vi "new Simulation1553Type.vi"(8 "error in":errorcluster, 11 "errorInjection configuration":T1 {"errorMessages" items=["Tagged", "Any"]; "state" items=["Off", "On", "Once", "External"]}) -> (0 "error out":errorcluster, 3 "new Simulation1553Type":refnum<k24>)   [LabVIEW 2020, in "Ballard_1553_Hardware_ni.lvlib"]
uses:
  Ballard_1553_Hardware_ni.lvlib
  C:/Users/Administrator/Desktop/GIT/Ballard-MIL-STD-1553-Custom-Device/Source/System Explorer/SubVIs/Parse XML Ballard/1.2/BTIXML_SerDes.dll
  Ballard-MIL-STD-1553-Custom-Device/Source/System Explorer/SubVIs/Parse XML Ballard/1.2/BTIXML_SerDes.dll
  _typedefs/channel1553_errorInjection_type.ctl
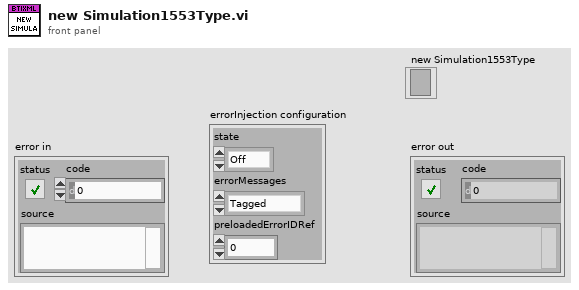
[diagram p1: front panel]
types:
  T1 = typedef "Ballard_1553_Hardware_ni.lvlib/channel1553_errorInjection_type.ctl" = cluster{"state":i32, "errorMessages":i32, "preloadedErrorIDRef":i32}
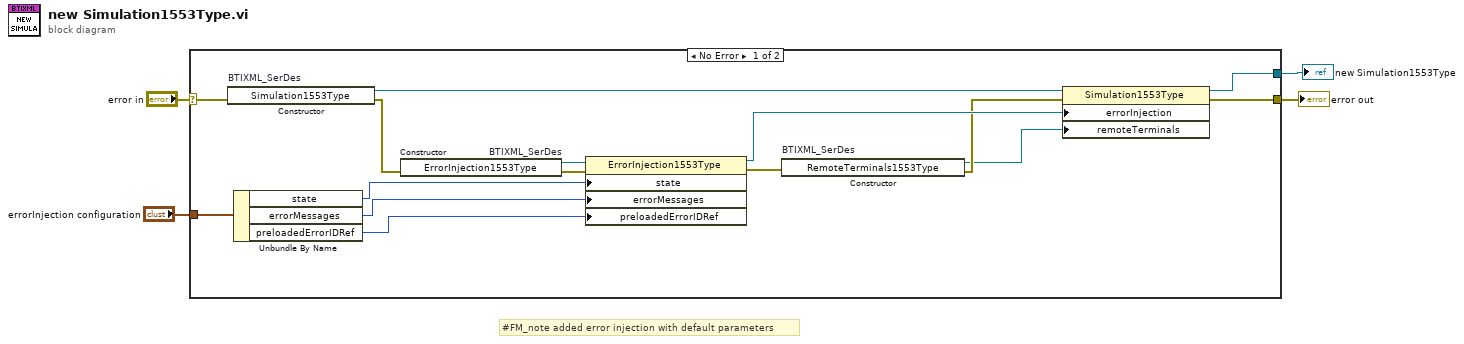
[diagram p0: block diagram]
diagram:
  # "#FM_note added error injection with default parameters"
  n1 = case shown="No Error" "error in" {
    selector: "error in" -> [w18 w20]
    tunnel: [w17 w20] -> w3
    tunnel: [w16 _] -> w1
    tunnel: "errorInjection configuration" -> [w12 _]
    frame No Error {
      n2 = constructor on="BTIXML_SerDes" class="Simulation1553Type"(error in=w18) -> (reference out=w19:refnum<k24>, error out=w13:errorcluster)  [unwired: 2 in, 1 out]
      n3 = Unbundle By Name(w12) -> ("state"=w11:i32, "errorMessages"=w10:i32, "preloadedErrorIDRef"=w9:i32)
      n4 = constructor on="BTIXML_SerDes" class="ErrorInjection1553Type"(error in=w13) -> (reference out=w15:refnum<k24>, error out=w14:errorcluster)  [unwired: 2 in, 1 out]
      n5 = property class="ErrorInjection1553Type"(reference=w15, error in=w14, "state"=w11, "errorMessages"=w10, "preloadedErrorIDRef"=w9) -> (reference out=w7:refnum<k24>, error out=w8:errorcluster)
      n6 = constructor on="BTIXML_SerDes" class="RemoteTerminals1553Type"(error in=w8) -> (reference out=w5:refnum<k24>, error out=w6:errorcluster)  [unwired: 2 in, 1 out]
      n7 = property class="Simulation1553Type"(reference=w19, error in=w6, "errorInjection"=w7, "remoteTerminals"=w5) -> (reference out=w16:refnum<k24>, error out=w17:errorcluster)
    }
    frame Error {
    }
  }
  "error out" <- w3
  "new Simulation1553Type" <- w1
